vi "Complex Single Tone Measurements.vi"() -> ()   [LabVIEW 2020]
doc: "This example measures the frequency and amplitude of the input complex signal. Unlike a real signal, the frequency of the complex signal can be negative. You can control the amplitude, frequency and noise level of the input signal. This example also shows the exported signal. <B>Signal to export</B> control specifies which signal to export. The sampling frequency of the input signal is 50 kHz in this example, <B>Frequency</B> must be in the range of (-25 kHz, 25 kHz)."
uses:
  <vilib>/measure/matone.llb/Extract Single Tone Information.vi
  <vilib>/measure/matone.llb/Extract Single Tone Information 1 Chan (CDB).vi
  <vilib>/measure/NI_MAPro.lvlib
panel:
  in  "Signal to export":T1(ring)=enum."input signal"
  out "Exported signal":waveform(dbl)[](graph)
  in  "Frequency":dbl=-235.0 format="%#.6g"
  in  "Amplitude":dbl=1.0000022000000006 format="%#.6g"
  in  "Stop":bool
  in  "Noise level (dB)":dbl(slide)=-3.6363636363636367
  out "Frequency detected":dbl
  out "Amplitude detected":dbl
  # "Overview: Demonstrates how to measure the frequency and amplitude of the input complex signal.\nRequirements: LabVIEW Full Development System\nInstructions: \n1. Run the VI. Note the agreement of the Input Signal values to the Detected Signal values even in a noisy signal.\n2. Change the Signal to export to detected signal to see only the detected tone in the signal.\n3. Click Stop to stop the VI."
  # "Input Signal"
  # "Detected Signal"
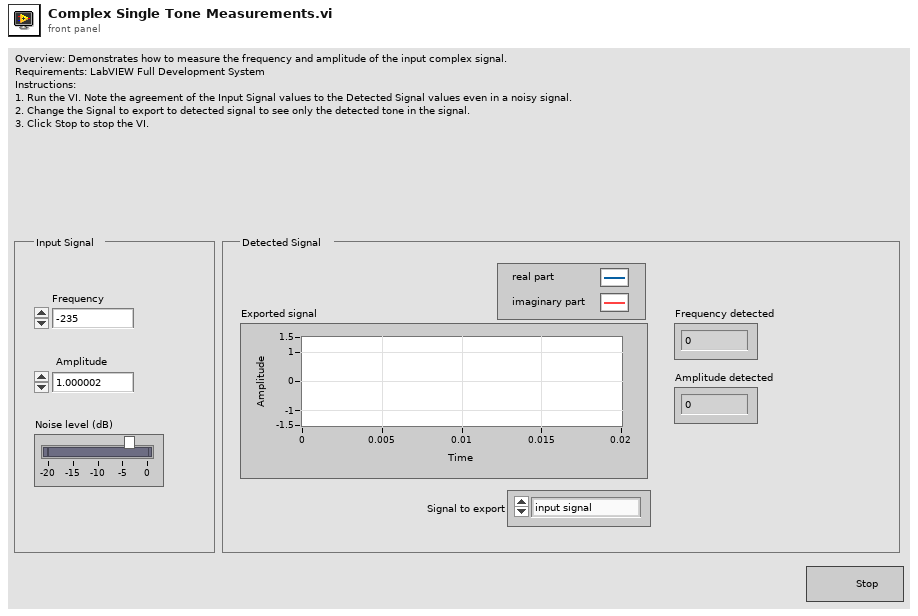
[diagram p1: front panel]
types:
  T1 = enum32{"none", "input signal", "detected signal", "residual signal"}
  T2 = cluster{"exported time signal":waveform(cdb), "exported spectrum (dB)":cluster{"f0":dbl, "df":dbl, "dB Spectrum (Hann)":dbl[]}}
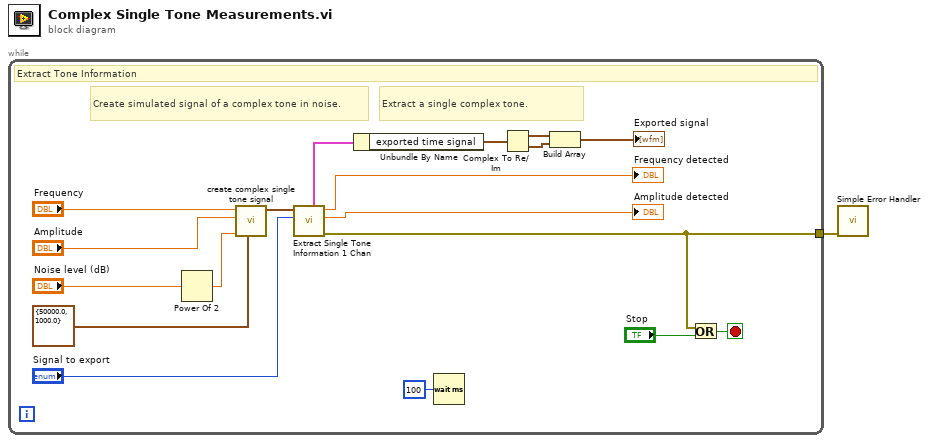
[diagram p0: block diagram]
diagram:
  n1 = while {
    tunnel: [w2] -> w1
    stop <- w3 stop-if-true
    # "Extract a single complex tone."
    # "Create simulated signal of a complex tone in noise."
    # "Extract Tone Information"
    n2 = Power Of 2(x="Noise level (dB)") -> (2^x=w11:dbl)
    n3 = call "create complex single tone signal.vi"("sampling info"=cluster{"Fs":dbl, "#s":dbl} {"Fs"=50000.0, "#s"=1000.0} ("Sampling info"), "Noise level"=w11, "amplitude"="Amplitude", "frequency (Hz)"="Frequency") -> ("complex waveform"=w14:waveform(cdb))  [unwired: 1 in, 6 out]
    n4 = call-poly "Extract Single Tone Information 1 Chan.vi"("export mode"="Signal to export", "time signal in"=w14) -> ("error out"=w2:errorcluster, "detected amplitude"=→"Amplitude detected":dbl, "detected frequency"=→"Frequency detected":dbl, "exported signals"=w12:T2)  [unwired: 2 in, 4 out]
    n5 = Unbundle By Name(w12) -> ("exported time signal"=w6:waveform(cdb))
    n6 = Wait (ms)(milliseconds to wait=u32 100) -> ()  [unwired: 1 out]
    n7 = Complex To Re/Im(x + iy=w6) -> (x=w8:waveform(dbl), y=w9:waveform(dbl))
    n8 = Build Array(w8, w9) -> (→"Exported signal":waveform(dbl)[])
    n9 = Or(x=w2, y="Stop") -> (x .or. y?=w3:bool)
  }
  n10 = call <vilib>:"Simple Error Handler.vi"("error in (no error)"=w1) -> ()  [unwired: 4 in, 5 out]
